vi "FilterCodes.vi"   [LabVIEW 2017, in "GPError.lvlib"]
doc: "Clears the error or warning on <B>Error in</B> if Code in <B>Error in</B> matches <B>Code to filter</B>.\n\nThis VI supports filtering appended errors, in which case it clears only those elements in the appended error collection that matches <B>Code to filter</B>.\n\n<B>Code filtered?</B> will be True only if <B>Error in</B> was filtered.\n\nThis VI is polymorphic, accepting either a single code or an array of codes to filter.\n\nSteen Schmidt\nGPower"
uses:
  GPError.lvlib
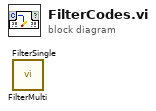
[diagram p0: block diagram]
diagram:
  n1 = call "FilterMulti.vi"() -> ()  [unwired: 10 in, 2 out]
  n2 = call "FilterSingle.vi"() -> ()  [unwired: 10 in, 2 out]
